vi "Snake_on_FPGA.vi"   [LabVIEW 2018]
uses:
  TypDefs/Player_Enum.ctl
  <vilib>/rvi/Emulation/niFpgaGetClockAttributes.vi
  <vilib>/rvi/Emulation/niFpgaSctlEmulationGetInTimedLoop.vi
  <vilib>/rvi/Emulation/niFpgaEmulationReportErrorSimple.vi
  Control/Global_GameOver.vi
  <vilib>/rvi/Emulation/niFpgaProcessEmulError.vi
  Game/Global_ScorePlayer1.vi
  Game/Global_ScorePlayer2.vi
  <vilib>/rvi/Emulation/niFpgaCriticalErrorInLSC.vi
panel:
  # "Snake on FPGA\nCreated by Pascal Heinen\nVI Technologies, Netherlands\nwww.vi-tech.nl\npascal@vi-tech.nl"
types:
  T1 = typedef "Player_Enum.ctl" = enum16{"Player 1", "Player 2"}
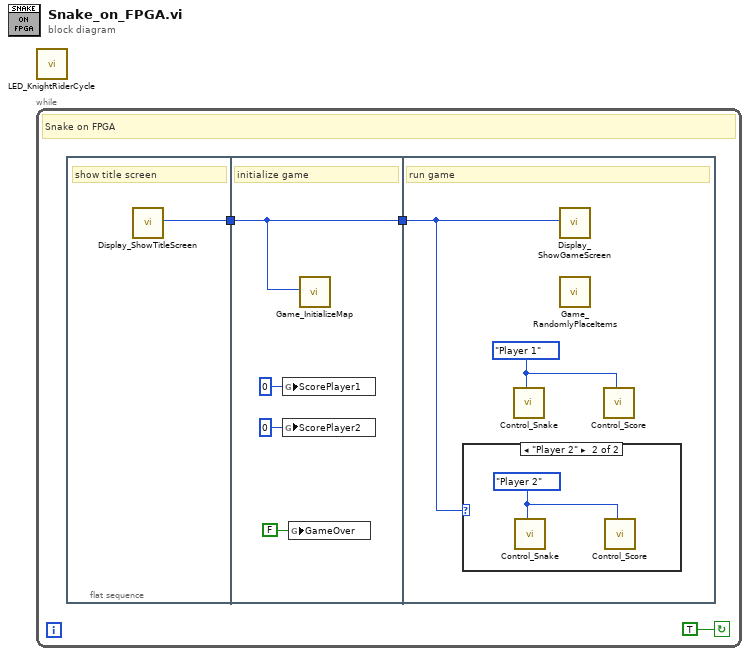
[diagram p0: block diagram]
diagram:
  n1 = call "LED_KnightRiderCycle.vi"() -> ()  [unwired: 12 in]
  n2 = while {
    stop <- TRUE continue-if-true
    # "Snake on FPGA"
    n3 = flat-sequence {
      tunnel: [w4] -> w2
      tunnel: w2 -> [w7]
      tunnel: [w7] -> w1
      tunnel: w1 -> [w10]
      frame #0 {
        # "show title screen"
        n4 = call "Display_ShowTitleScreen.vi"() -> ("SelectedNrOfPlayers"=w4:T1)  [unwired: 19 in]
      }
      frame #1 {
        # "initialize game"
        n5 = global write "Global_ScorePlayer1.vi" "ScorePlayer1"(u16 0 ("ScorePlayer1")) -> ()
        n6 = global write "Global_ScorePlayer2.vi" "ScorePlayer2"(u16 0 ("ScorePlayer2")) -> ()
        n7 = global write "Global_GameOver.vi" "GameOver"(FALSE ("Stop")) -> ()
        n8 = call "Game_InitializeMap.vi"("NrOfPlayers"=w7) -> ()  [unwired: 19 in]
      }
      frame #2 {
        w9 = Player_Enum."Player 1" ("Player")
        # "run game"
        n9 = case shown="\"Player 2\"" w10 {
          frame "Player 1" {
          }
          frame "Player 2" {
            w11 = Player_Enum."Player 2" ("Player")
            n10 = call "Control_Snake.vi"("Player"=w11) -> ()  [unwired: 19 in]
            n11 = call "Control_Score.vi"("Player"=w11) -> ()  [unwired: 19 in]
          }
        }
        n12 = call "Control_Snake.vi"("Player"=w9) -> ()  [unwired: 19 in]
        n13 = call "Display_ShowGameScreen.vi"("Player"=w10) -> ()  [unwired: 19 in]
        n14 = call "Game_RandomlyPlaceItems.vi"() -> ()  [unwired: 20 in]
        n15 = call "Control_Score.vi"("Player"=w9) -> ()  [unwired: 19 in]
      }
    }
  }
